vi "simArbSignal_coolDown.vi"(7 "dt":dbl=5.0 format="%0.6f", 8 "error in (no error)":errorcluster, 9 "Reset":bool, 10 "Next Value":bool=TRUE, 11 "Data":dbl[][](array[numeric])=[[0.0, 5.0, 10.0, 15.0, 20.0, 25.0, 30.0, 35.0, 40.0, 45.0, 50.0, 55.0, 60.0, 65.0, 70.0, 75.0, 80.0, 85.0, 90.0, 95.0, 100.0, 105.0, 110.0, 115.0, 120.0, 125.0, 130.0, 135.0, 140.0, 145.0, 150.0, 155.0, 160.0, 165.0, 170.0, 175.0, 180.0, 185.0, 190.0, 195.0, 200.0, 205.0, 210.0, 215.0, 220.0, 225.0, 230.0, 235.0, 240.0, 245.0, 250.0, 255.0, 260.0, 265.0, 270.0, 275.0, 280.0, 285.0, 290.0, 295.0, 300.0, 305.0, 310.0, 315.0, 320.0, 325.0, 330.0, 335.0, 340.0, 345.0, 350.0, 355.0, 360.0, 365.0, 370.0, 375.0, 380.0, 385.0, 390.0, 395.0, 400.0, 405.0, 410.0, 415.0, 420.0, 425.0, 430.0, 435.0, 440.0, 445.0, 450.0, 455.0, 460.0, 465.0, 470.0, 475.0, 480.0, 485.0, 490.0, 495.0, 500.0, 505.0, 510.0, 515.0, 520.0, 525.0, 530.0, 535.0, 540.0, 545.0, 550.0, 555.0, 560.0, 565.0, 570.0, 575.0, 580.0, 585.0, 590.0, 595.0, 600.0, 605.0, 610.0, 615.0, 620.0, 625.0, 630.0, 635.0, 640.0, 645.0, 650.0, 655.0, 660.0, 665.0, 670.0, 675.0, 680.0, 685.0, 690.0, 695.0, 700.0, 705.0, 710.0, 715.0, 720.0, 725.0, 730.0, 735.0, 740.0, 745.0, 750.0, 755.0, 760.0, 765.0, 770.0, 775.0, 780.0, 785.0, 790.0, 795.0, 800.0, 805.0, 810.0, 815.0, 820.0, 825.0, 830.0, 835.0, 840.0, 845.0, 850.0, 855.0, 860.0, 865.0, 870.0, 875.0, 880.0, 885.0, 890.0, 895.0, 900.0, 905.0, 910.0, 915.0, 920.0, 925.0, 930.0, 935.0, 940.0, 945.0, 950.0, 955.0, 960.0, 965.0, 970.0, 975.0, 980.0, 985.0, 990.0, 995.0, 1000.0, 1005.0, 1010.0, 1015.0, 1020.0, 1025.0, 1030.0, 1035.0, 1040.0, 1045.0, 1050.0, 1055.0, 1060.0, 1065.0, 1070.0, 1075.0, 1080.0, 1085.0, 1090.0, 1095.0, 1100.0, 1105.0, 1110.0, 1115.0, 1120.0, 1125.0, 1130.0, 1135.0, 1140.0, 1145.0, 1150.0, 1155.0, 1160.0, 1165.0, 1170.0, 1175.0, 1180.0, 1185.0, 1190.0, 1195.0, 1200.0, 1205.0, 1210.0, 1215.0, 1220.0, 1225.0, 1230.0, 1235.0, 1240.0, 1245.0, 1250.0, 1255.0, 1260.0, 1265.0, 1270.0, 1275.0, 1280.0, 1285.0, 1290.0, 1295.0, 1300.0, 1305.0, 1310.0, 1315.0, 1320.0, 1325.0, 1330.0, 1335.0, 1340.0, 1345.0, 1350.0, 1355.0, 1360.0, 1365.0, 1370.0, 1375.0, 1380.0, 1385.0, 1390.0, 1395.0, 1400.0, 1405.0, 1410.0, 1415.0, 1420.0, 1425.0, 1430.0, 1435.0, 1440.0, 1445.0, 1450.0, 1455.0, 1460.0, 1465.0, 1470.0, 1475.0, 1480.0, 1485.0, 1490.0, 1495.0, 1500.0, 1505.0, 1510.0, 1515.0, 1520.0, 1525.0, 1530.0, 1535.0, 1540.0, 1545.0, 1550.0, 1555.0, 1560.0, 1565.0, 1570.0, 1575.0, 1580.0, 1585.0, 1590.0, 1595.0, 1600.0, 1605.0, 1610.0, 1615.0, 1620.0, 1625.0, 1630.0, 1635.0, 1640.0, 1645.0, 1650.0, 1655.0, 1660.0, 1665.0, 1670.0, 1675.0, 1680.0, 1685.0, 1690.0, 1695.0, 1700.0, 1705.0, 1710.0, 1715.0, 1720.0, 1725.0, 1730.0, 1735.0, 1740.0, 1745.0, 1750.0, 1755.0, 1760.0, 1765.0, 1770.0, 1775.0, 1780.0, 1785.0, 1790.0, 1795.0, 1800.0, 1805.0], [0.001, 0.09989040826998175, 0.10291343875305299, 0.10582849186251818, 0.10874354497198305, 0.11165859808144823, 0.1145736511909131, 0.11748870430037828, 0.12040375740984316, 0.12331881051930833, 0.1262338636287732, 0.1291489167382384, 0.13206396984770327, 0.13497902295716846, 0.13789407606663362, 0.1408091291760985, 0.1437241822855637, 0.14663923539502854, 0.14955428850449373, 0.15246934161395861, 0.1553843947234238, 0.15829944783288866, 0.16121450094235384, 0.16412955405181873, 0.1670446071612839, 0.16995966027074907, 0.17287471338021396, 0.17578976648967914, 0.17870481959914403, 0.1816198727086092, 0.18453492581807407, 0.18744997892753923, 0.1903650320370041, 0.1932800851464693, 0.19619513825593415, 0.19911019136539937, 0.20202524447486422, 0.2049402975843294, 0.20785535069379457, 0.21077040380325945, 0.21368545691272464, 0.2166005100221895, 0.2195155631316547, 0.22243061624111957, 0.22534566935058475, 0.2282607224600496, 0.2311757755695148, 0.23409082867897968, 0.23700588178844487, 0.23992093489790972, 0.2428359880073749, 0.2457510411168401, 0.24866609422630498, 0.25158114733577014, 0.254496200445235, 0.2574112535547002, 0.26032630666416506, 0.2632413597736303, 0.2661564128830951, 0.2690714659925603, 0.2719865191020252, 0.27490157221149036, 0.2778166253209555, 0.2807316784304204, 0.2836467315398856, 0.28656178464935045, 0.28947683775881566, 0.29239189086828055, 0.2953069439777457, 0.2982219970872106, 0.30113705019667575, 0.30405210330614063, 0.3069671564156058, 0.309882209525071, 0.3127972626345359, 0.3157123157440007, 0.31862736885346593, 0.32154242196293115, 0.324457475072396, 0.32737252818186113, 0.33028758129132607, 0.33320263440079123, 0.33611768751025606, 0.3390327406197213, 0.34194779372918616, 0.3448628468386513, 0.3477778999481162, 0.3506929530575814, 0.3536080061670466, 0.3565230592765114, 0.35943811238597656, 0.3623531654954415, 0.36526821860490666, 0.3681832717143715, 0.37109832482383676, 0.3740133779333016, 0.37692843104276674, 0.3798434841522317, 0.38275853726169684, 0.385673590371162, 0.3885886434806268, 0.39150369659009177, 0.3944187496995569, 0.3973338028090221, 0.400248855918487, 0.4031639090279522, 0.406078962137417, 0.4089940152468823, 0.4119090683563471, 0.41482412146581227, 0.4177391745752774, 0.42065422768474237, 0.4235692807942075, 0.42648433390367235, 0.4293993870131376, 0.43231444012260245, 0.4352294932320676, 0.43814454634153255, 0.4410595994509977, 0.44397465256046253, 0.4468897056699277, 0.44980475877939297, 0.4527198118888578, 0.4556348649983226, 0.4585499181077879, 0.46146497121725305, 0.4643800243267179, 0.46729507743618304, 0.470210130545648, 0.47312518365511314, 0.47604023676457796, 0.47895528987404323, 0.4818703429835084, 0.4847853960929732, 0.48770044920243816, 0.4906155023119033, 0.4935305554213685, 0.4964456085308333, 0.4993606616402986, 0.5022757147497634, 0.5051907678592286, 0.5081058209686935, 0.5110208740781587, 0.5139359271876235, 0.5168509802970886, 0.5197660334065536, 0.5226810865160187, 0.5255961396254839, 0.5285111927349488, 0.5314262458444137, 0.5343412989538788, 0.537256352063344, 0.5401714051728089, 0.5430864582822741, 0.5460015113917389, 0.5489165645012042, 0.551831617610669, 0.5547466707201342, 0.5576617238295993, 0.5605767769390643, 0.5634918300485291, 0.5664068831579943, 0.5693219362674595, 0.5722369893769244, 0.5751520424863895, 0.5780670955958545, 0.5809821487053196, 0.5838972018147844, 0.5868122549242496, 0.5897273080337149, 0.5926423611431797, 0.5955574142526445, 0.5984724673621098, 0.601387520471575, 0.6043025735810398, 0.6072176266905049, 0.6101326797999699, 0.613047732909435, 0.6159627860188999, 0.618877839128365, 0.62179289223783, 0.6247079453472951, 0.62762299845676, 0.6305380515662252, 0.6334531046756904, 0.6363681577851552, 0.6392832108946201, 0.6421982640040853, 0.6451133171135505, 0.6480283702230153, 0.6509434233324806, 0.6538584764419454, 0.6567735295514106, 0.6596885826608755, 0.6626036357703406, 0.6655186888798058, 0.6684337419892706, 0.6713487950987356, 0.6742638482082007, 0.6771789013176659, 0.6800939544271308, 0.683009007536596, 0.6859240606460608, 0.6888391137555261, 0.6917541668649909, 0.6946692199744561, 0.6975842730839212, 0.7004993261933862, 0.703414379302851, 0.7063294324123162, 0.7092444855217814, 0.7121595386312463, 0.7150745917407111, 0.7179896448501764, 0.7209046979596415, 0.7238197510691063, 0.7267348041785715, 0.7296498572880364, 0.7325649103975016, 0.7354799635069664, 0.7383950166164317, 0.7413100697258969, 0.7442251228353617, 0.7471401759448266, 0.7500552290542918, 0.7529702821637569, 0.7558853352732218, 0.758800388382687, 0.7617154414921519, 0.764630494601617, 0.767545547711082, 0.7704606008205471, 0.7733756539300123, 0.7762907070394771, 0.779205760148942, 0.7821208132584072, 0.7850358663678724, 0.7879509194773373, 0.7908659725868025, 0.7937810256962673, 0.7966960788057325, 0.7996111319151974, 0.7942258713080907, 0.7875629025890629, 0.7808999338700353, 0.7742369651510078, 0.7675739964319803, 0.7609110277129525, 0.7542480589939249, 0.7475850902748974, 0.7409221215558699, 0.7342591528368421, 0.7275961841178145, 0.720933215398787, 0.7142702466797595, 0.7076072779607316, 0.700944309241704, 0.6942813405226765, 0.687618371803649, 0.6809554030846212, 0.6742924343655936, 0.6676294656465661, 0.6609664969275386, 0.6543035282085108, 0.6476405594894832, 0.6409775907704557, 0.6343146220514282, 0.6276516533324004, 0.6209886846133728, 0.6143257158943453, 0.6076627471753178, 0.6009997784562899, 0.5943368097372623, 0.5876738410182348, 0.5810108722992073, 0.5743479035801798, 0.5676849348611519, 0.5610219661421244, 0.5543589974230969, 0.5476960287040691, 0.5410330599850415, 0.534370091266014, 0.5277071225469865, 0.5210441538279589, 0.514381185108931, 0.5077182163899036, 0.5010552476708761, 0.4943922789518482, 0.4877293102328206, 0.4810663415137931, 0.47440337279476563, 0.4677404040757381, 0.4610774353567102, 0.4544144666376827, 0.4477514979186552, 0.4410885291996273, 0.43442556048059977, 0.4277625917615723, 0.4210996230425448, 0.41443665432351723, 0.40777368560448934, 0.40111071688546185, 0.39444774816643435, 0.38778477944740647, 0.3811218107283789, 0.3744588420093514, 0.3677958732903239, 0.3611329045712964, 0.3544699358522685, 0.347806967133241, 0.3411439984142135, 0.3344810296951856, 0.32781806097615807, 0.32115509225713057, 0.3144921235381031, 0.3078291548190755, 0.30116618610004764, 0.29450321738102014, 0.28784024866199265, 0.2811772799429647, 0.2745143112239372, 0.2678513425049097, 0.2611883737858822, 0.2545254050668547, 0.2478624363478268, 0.2411994676287993, 0.2345364989097718, 0.2278735301907443, 0.2212105614717167, 0.21454759275268886, 0.20788462403366137, 0.20122165531463387, 0.19455868659560593, 0.18789571787657844, 0.18123274915755094, 0.17456978043852334, 0.16790681171949584, 0.161243843000468, 0.15458087428144052, 0.1479179055624129, 0.14125493684338508, 0.13459196812435759, 0.1279289994053301, 0.12126603068630248, 0.11460306196727499, 0.10794009324824716, 0.10127712452921966, 0.09461415581019206, 0.08795118709116423, 0.08128821837213673, 0.07462524965310924, 0.06796228093408163, 0.061299312215054136, 0.05463634349602631, 0.04797337477699881, 0.041310406057971205, 0.034647437338943377, 0.02798446861991588, 0.021321499900888385, 0.014658531181860779, 0.007995562462833283, 0.0013325937438054547]]) -> (0 "error out":errorcluster, 2 "Data Valid":bool, 3 "Signal":dynamicdata(graph)=[{"t0"=timestamp(0 s since 1904-01-01), "dt"=5.0, "Y"=array[362 elements], "attributes"=variant("NI_ChannelName"=variant(string "Signal"))}])   [LabVIEW 2017]
doc: "Simulates a signal that you define.\n--------------------\n\nThis Express VI is configured as follows:\n\nMode: Packet (The whole waveform each run)\nCurve Specifications: Hold last value"
panel:
  in  "Repeat":bool
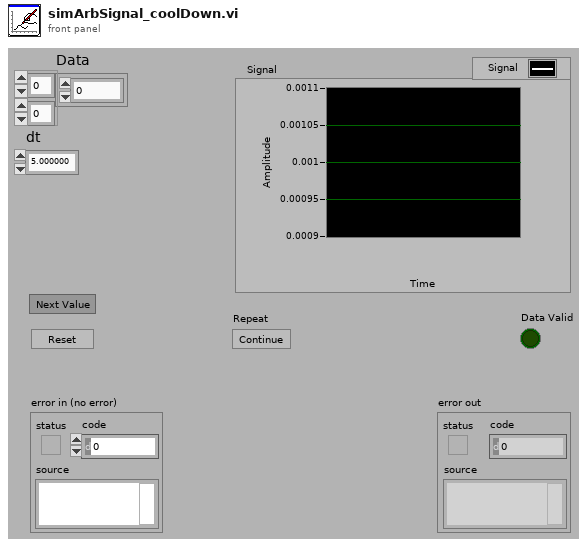
[diagram p1: front panel]
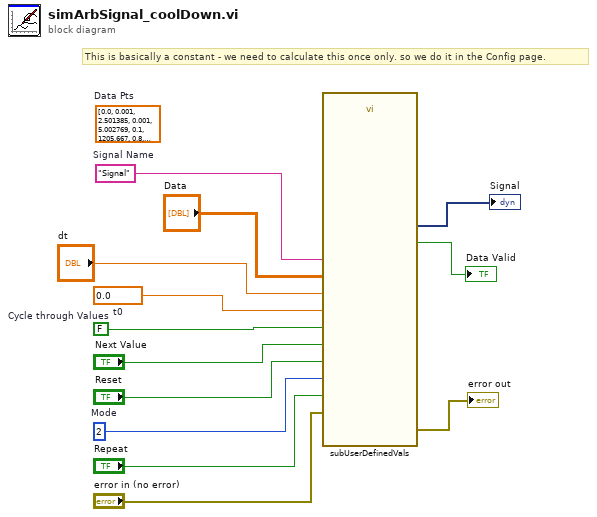
[diagram p0: block diagram]
diagram:
  (unwired) dbl[][] [[0.0, 0.001], [2.501385, 0.001], [5.002769, 0.1], [1205.667, 0.8], [1806.0, 0.0], [1806.5, 0.0]]  # Data Pts
  w4 = 2  # Mode
  w6 = FALSE  # Cycle through Values
  w7 = 0.0  # t0
  w13 = "Signal"  # Signal Name
  # "This is basically a constant - we need to calculate this once only. so we do it in the Config page."
  n1 = call <vilib>:"subUserDefinedVals.vi"("t0"=w7, "Next Value"="Next Value", "Mode"=w4, "dt"="dt", "error in (no error)"="error in (no error)", "Array"="Data", "Signal Name"=w13, "Cycle through Values"=w6, "Repeat"="Repeat", "Reset"="Reset") -> ("Signal"=→"Signal":dynamicdata, "error out"=→"error out":errorcluster, "Data Valid"=→"Data Valid":bool)  [unwired: 3 in]
